vi "Select Channel.vi"(8 "error in (no error)":errorcluster, 9 "Table Name":string, 10 "Select Channels":string[](array[string]), 11 "Data Loader in":refnum<class "Data Loader.lvclass">) -> (0 "error out":errorcluster, 3 "Data Loader out":refnum<class "Data Loader.lvclass">)   [LabVIEW 2020, in "Data Loader.lvlib" / "Data Loader.lvclass"]
uses:
  Data Loader.lvclass
  Data Loader.lvclass/Data Loader.ctl
  Data Types/Abstrut Data/Abstruct Data Type.lvclass/Abstruct Data Type.ctl
  MVVM Framework/MVVM Abstruct Model/MVVM Abstruct Model/MVVM Abstruct Model.lvclass/MVVM Abstruct Model.ctl
  Views/Data Interface/Data Interface Messages/Update Data Msg/Update Data Msg.lvclass/Update Data Msg.ctl
  <vilib>/ActorFramework/Message Enqueuer/Message Enqueuer.lvclass/Message Enqueuer.ctl
  MVVM Framework/MVVM Abstruct Model/MVVM Abstruct Model/Accessor/Read ActorMap-Views.vi
  <vilib>/ActorFramework/Message Enqueuer/Enqueue.vi
  Views/Data Interface/Data Interface Messages/Update Data Msg/Update Data Msg.lvclass
  C:/Program Files (x86)/National Instruments/LabVIEW 2020/vi.lib/ActorFramework/Message/Message.lvclass
  <vilib>/ActorFramework/Message Priority Queue/Priority Enqueue.vi
  <vilib>/ActorFramework/Message Enqueuer/Message Enqueuer.lvclass
  Depden On/ActorMap/ActorMap.lvclass
  Data Types/Abstrut Data/Abstruct Data Type.lvclass
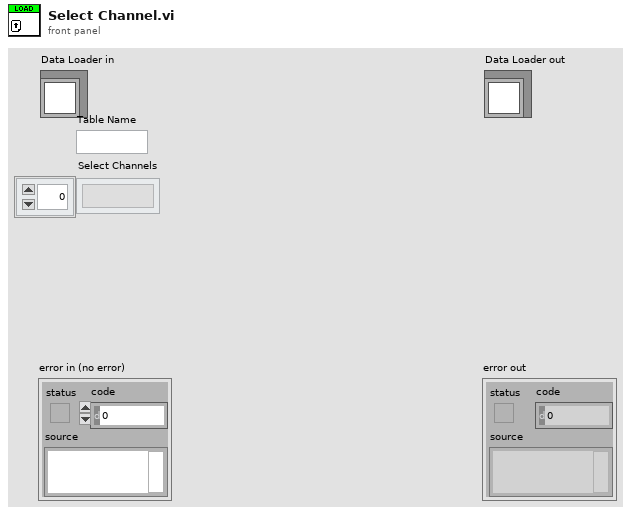
[diagram p1: front panel]
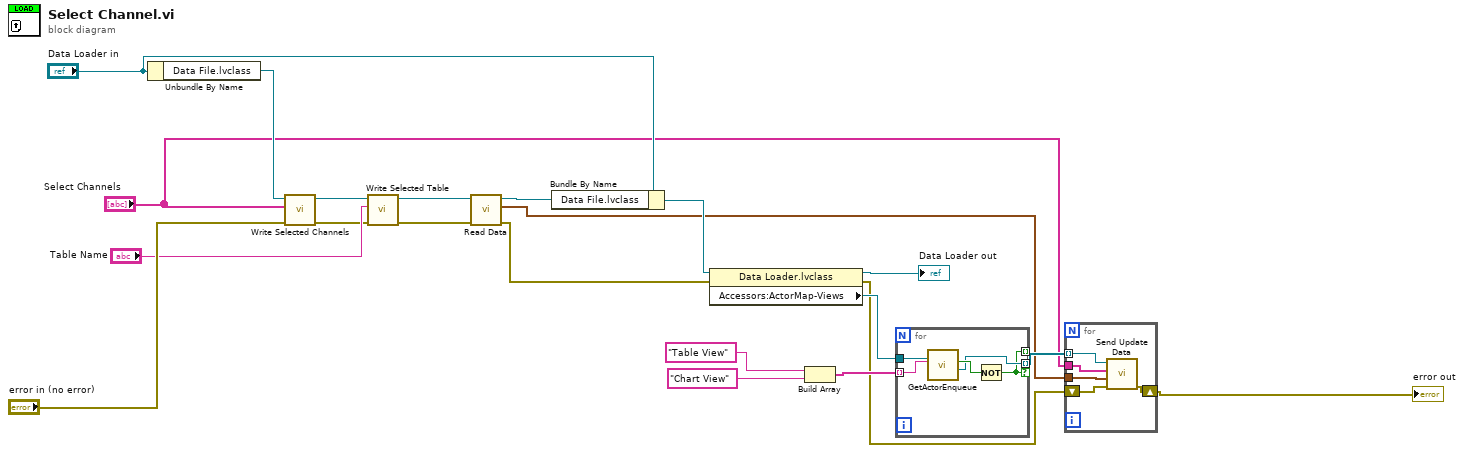
[diagram p0: block diagram]
diagram:
  n1 = Unbundle By Name("Data Loader in") -> ("Data File.lvclass"=w19:refnum<class "Abstruct Data Type.lvclass">)
  n2 = call "Write Selected Channels.vi"("error in (no error)"="error in (no error)", "Selected Channels"="Select Channels", "Abstruct Data Type in"=w19) -> ("error out"=w2:errorcluster, "Abstruct Data Type out"=w5:refnum<class "Abstruct Data Type.lvclass">)  [unwired: 7 in]
  n3 = call "Write Selected Table.vi"("error in (no error)"=w2, "Selected Table"="Table Name", "Abstruct Data Type in"=w5) -> ("error out"=w1:errorcluster, "Abstruct Data Type out"=w4:refnum<class "Abstruct Data Type.lvclass">)  [unwired: 7 in]
  n4 = call-dynamic "Read Data.vi"("error in (no error)"=w1, "Abstruct Data Type in"=w4) -> ("error out"=w6:errorcluster, "data"=w10:waveform(dbl)[], "Abstruct Data Type out"=w20:refnum<class "Abstruct Data Type.lvclass">)  [unwired: 7 in]
  n5 = Bundle By Name(cluster="Data Loader in", "Data File.lvclass"=w20) -> (w17:refnum<class "Data Loader.lvclass">)
  n6 = property class="Data Loader.lvclass"(reference=w17, error in=w6) -> (reference out=→"Data Loader out":refnum<class "Data Loader.lvclass">, error out=w8:errorcluster, "Accessors:ActorMap-Views"=w15:refnum<class "ActorMap.lvclass">)
  n7 = Build Array("Table View", "Chart View") -> (w13:string[])
  n8 = for {
    tunnel: w15 -> [w26]
    tunnel: w13 -> [w25] mode=indexing
    tunnel: [w22] -> _ mode=indexing
    tunnel: [w23] -> w11 mode=indexing if=w22
    n9 = call "GetActorEnqueue.vi"("name"=w25, "ActorMap in"=w26) -> ("Enqueue"=w23:refnum<class "Message Enqueuer.lvclass">, "key not found?"=w24:bool)  [unwired: 6 in, 2 out]
    n10 = Not(x=w24) -> (.not. x?=w22:bool)
  }
  n11 = for {
    tunnel: w11 -> [w31] mode=indexing
    tunnel: w10 -> [w30]
    tunnel: "Select Channels" -> [w29]
    shift-right: [w27] -> w7
    shift-left: w8 -> [w28]
    n12 = call "Send Update Data.vi"("error in (no error)"=w28, "data"=w30, "Channel Names"=w29, "Message Enqueuer"=w31) -> ("error out"=w27:errorcluster)  [unwired: 6 in, 1 out]
  }
  "error out" <- w7
